vi "ValidateCommand.vi"(4 "input message 4":string) -> (0 "MECH":string, 1 "CMD":string, 2 "PARAM":string, 3 "err_out":bool)   [LabVIEW 2012]
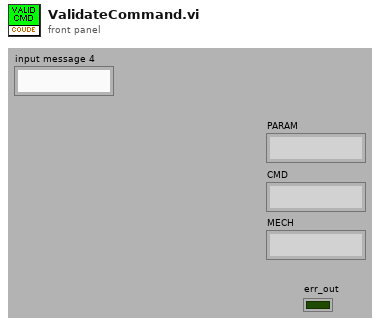
[diagram p1: front panel]
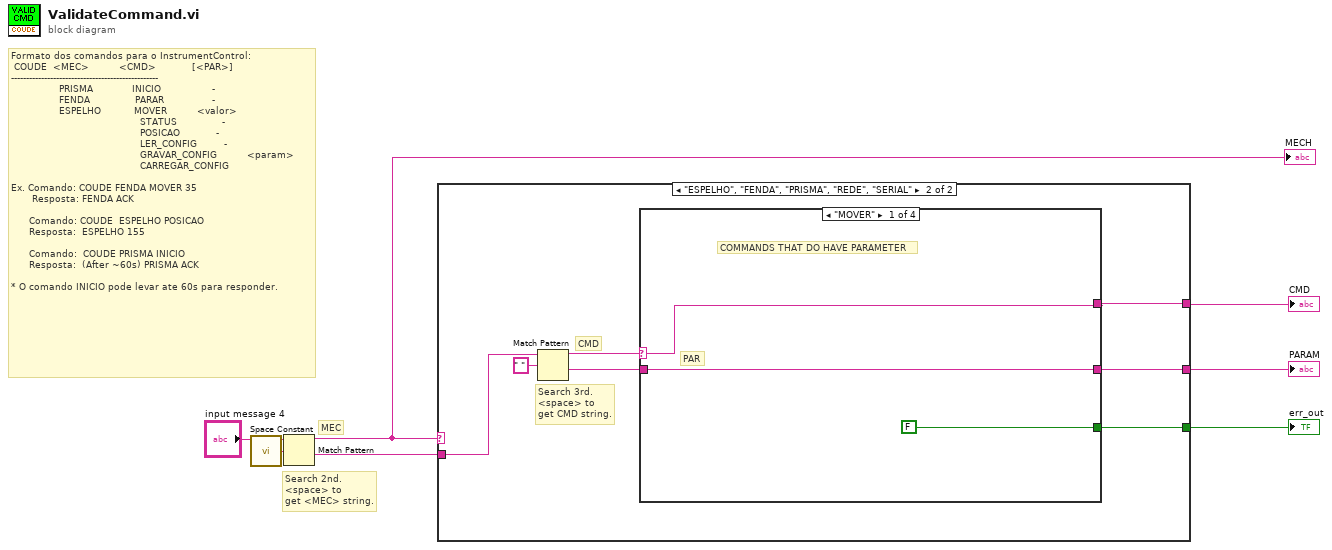
[diagram p0: block diagram]
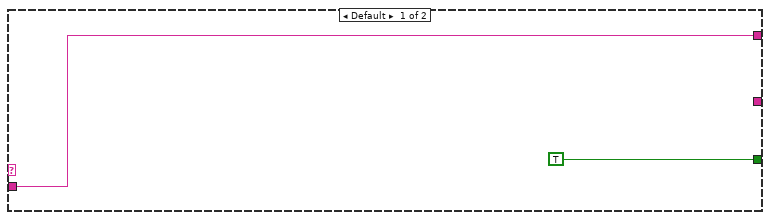
[diagram p2: hidden frame]
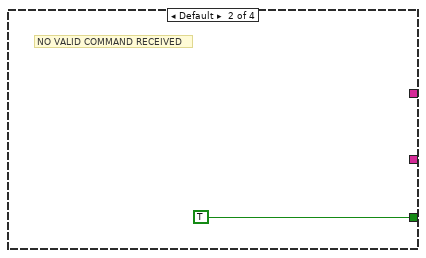
[diagram p3: hidden frame]
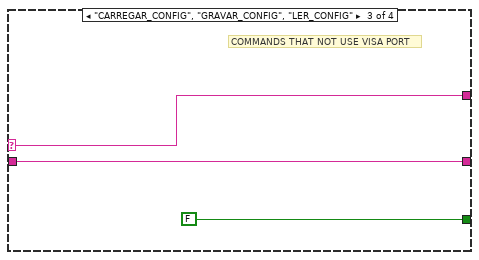
[diagram p4: hidden frame]
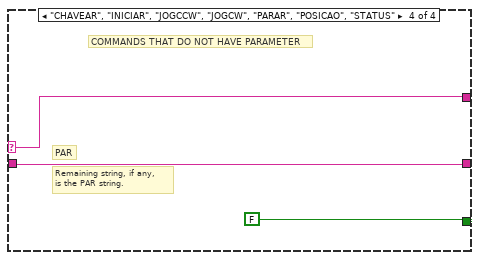
[diagram p5: hidden frame]
diagram:
  # "Formato dos comandos para o InstrumentControl:\n COUDE  <MEC>          <CMD>            [<PAR>]\n-------------------------------------------------\n                PRISMA             INICIO                 -\n                FENDA               PARAR                - \n                ESPELHO           MOVER          <valor>                 \n                                           STATUS               -\n                                           POSICAO            -\n                                           LER_CONFIG         -\n                                           GRAVAR_CONFIG          <param>\n                                           CARREGAR_CONFIG\n          \nEx. Comando: COUDE FENDA MOVER 35\n       Resposta: FENDA ACK\n    \n      Comando: COUDE  ESPELHO POSICAO\n      Resposta:  ESPELHO 155\n\n      Comando:  COUDE PRISMA INICIO\n      Resposta:  (After ~60s) PRISMA ACK \n\n* O comando INICIO pode levar ate 60s para responder."
  # "MEC"
  # "Search 2nd.\n<space> to\nget <MEC> string."
  n1 = call <vilib>:"Space Constant.vi"() -> ("String"=w7:string)
  n2 = Match Pattern(string="input message 4", regular expression=w7) -> (before substring=w1:string, after substring=w3:string)  [unwired: 3 out]
  "MECH" <- w1
  n3 = case shown="\"ESPELHO\", \"FENDA\", \"PRISMA\", \"REDE\", \"SERIAL\"" w1 {
    tunnel: [_ w15] -> w6
    tunnel: [w8 w14] -> w4
    tunnel: w3 -> [w8 w16]
    tunnel: [TRUE w11] -> w2
    frame Default {
    }
    frame "ESPELHO", "FENDA", "PRISMA", "REDE", "SERIAL" {
      # "CMD"
      # "Search 3rd.\n<space> to\nget CMD string."
      n4 = Match Pattern(string=w16, regular expression=" ") -> (before substring=w13:string, after substring=w12:string)  [unwired: 3 out]
      n5 = case shown="\"MOVER\"" w13 {
        selector: w13 -> [w19 _ w23 w26]
        tunnel: [w18 _ w22 w25] -> w15
        tunnel: [w19 _ w23 w26] -> w14
        tunnel: w12 -> [w18 _ w22 w25]
        tunnel: [FALSE TRUE FALSE FALSE] -> w11
        frame "MOVER" {
          # "PAR"
          # "COMMANDS THAT DO HAVE PARAMETER"
        }
        frame Default {
          # "NO VALID COMMAND RECEIVED"
        }
        frame "CARREGAR_CONFIG", "GRAVAR_CONFIG", "LER_CONFIG" {
          # "COMMANDS THAT NOT USE VISA PORT"
        }
        frame "CHAVEAR", "INICIAR", "JOGCCW", "JOGCW", "PARAR", "POSICAO", "STATUS" {
          # "COMMANDS THAT DO NOT HAVE PARAMETER"
          # "Remaining string, if any,\nis the PAR string."
          # "PAR"
        }
      }
    }
  }
  "PARAM" <- w6
  "CMD" <- w4
  "err_out" <- w2
